vi "Autonomous Independent.vi"() -> ()   [LabVIEW 2017]
doc: "This VI is called when autonomous begins, and will automatically be terminated when autonomous ends. You can carry out timed or sensor driven robot movement independently without needing to return to the caller."
uses:
  <vilib>/Rock Robotics/WPI/Solenoid/WPI_SolenoidValue.ctl
  <vilib>/Rock Robotics/WPI/SafetyOutput/WPI_SafetyOutputConfigMenu.ctl
  <vilib>/Rock Robotics/WPI/Utilities/WPI_GetSetVariantRefNum.vi
  <vilib>/Rock Robotics/Network Tables/NT Read String.vi
  <vilib>/Rock Robotics/Network Tables/NT Write Numeric Array.vi
  <vilib>/Rock Robotics/WPI/Solenoid/WPI_SolenoidSetEnum.vi
  <vilib>/Rock Robotics/Network Tables/NT Read Numeric Array.vi
  <vilib>/Rock Robotics/Network Tables/NT Read Number.vi
  Robot Global Data.vi
  <vilib>/Rock Robotics/WPI/RobotDrive/WPI_RobotDriveArcadeDrive_Standard(NoSaturation).vi
panel:
  in  "Gear and B":dbl[](array[numeric])=[79.0, -39.5, 48.0, 160.0]
  in  "Drive Forward":dbl[](array[numeric])=[102.0, 0.0, 0.0, 0.0]
  in  "Station 3 Distances":dbl[](array[numeric])=[108.0, 10.0, -10.0, 20.0]
  in  "Station 1 Distances":dbl[](array[numeric])=[48.0, 24.0, -24.0, 96.0]
  in  "Station 2 Distances":dbl[](array[numeric])=[90.0, -48.0, 48.0, 120.0]
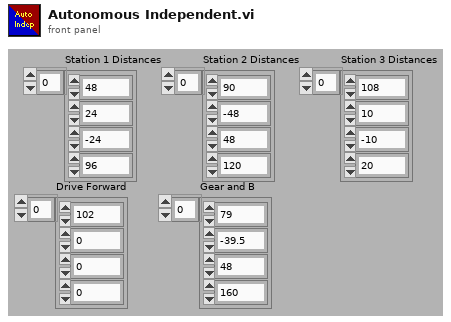
[diagram p1: front panel]
types:
  T1 = typedef "WPI_SolenoidValue.ctl" = enum16{"Off", "On", "Forward", "Reverse"}
  T2 = typedef "WPI_SolenoidDevRef.ctl" = cluster{"DevStatus":errorcluster, "Pneumatics Control Module":u8, "Forward Solenoid Channel":T3, "Reverse Solenoid Channel":T3}
  T3 = typedef "WPI_SolenoidChannel.ctl" = enum8{"Solenoid 0", "Solenoid 1", "Solenoid 2", "Solenoid 3", "Solenoid 4", "Solenoid 5", "Solenoid 6", "Solenoid 7", "Invalid"}
  T4 = typedef "WPI_JoystickDevRef.ctl" = cluster{"Device":T5}
  T5 = typedef "WPI_JoystickDeviceEnum.ctl" = enum16{"USB 0", "USB 1", "USB 2", "USB 3", "USB 4", "USB 5"}
  T6 = cluster{"Numeric Array":dbl[], "Numeric":dbl, "Numeric":dbl, "Numeric":dbl}
  T7 = cluster{"Numeric Array":dbl[], "Numeric":dbl, "Numeric":dbl}
  T8 = typedef "WPI_SafetyOutputConfigMenu.ctl" = enum16{"Enable", "Disable"}
  T9 = typedef "WPI_RobotDriveDevRef.ctl" = cluster{"DevStatus":errorcluster, "Motors[]":T10[], "Square Inputs":bool, "Max Output":dbl}
  T10 = typedef "WPI_MotorControlDeviceRef.ctl" = cluster{"DeviceStatus":errorcluster, "Type":T11, "PWM":cluster{"PWM Channel":T12, "DeadBand":T13}, "CAN":cluster{"Device Number":u8, "SetOutput VI Ref":variant, "GetOutput VI Ref":variant, "Enable VI Ref":variant, "Disable VI Ref":variant, "Data":variant}, "Invert":bool, "DIO PWM":cluster{"PWM \"Enable\" Channel":T12, "DIOChannel":T14, "PWM Rate":dbl}}
  T11 = typedef "WPI_MotorControlType.ctl" = enum16{"PWM", "CAN", "DIO PWM"}
  T12 = typedef "FPGA_DIOPWMChannel.ctl" = enum8{"PWM 0", "PWM 1", "PWM 2", "PWM 3", "PWM 4", "PWM 5", "PWM 6", "PWM 7", "PWM 8", "PWM 9", "PWM MXP 0", "PWM MXP 1", "PWM MXP 2", "PWM MXP 3", "PWM MXP 4", "PWM MXP 5", "PWM MXP 6", "PWM MXP 7", "PWM MXP 8", "PWM MXP 9", "Invalid"}
  T13 = typedef "WPI_PWMDeadband.ctl" = cluster{"Name":string, "maxPositivePwm":i32, "minPositivePwm":i32, "centerPwm":i32, "maxNegativePwm":i32, "minNegativePwm":i32, "angularRange":u16}
  T14 = typedef "FPGA_DIOChannel.ctl" = enum8{"DIO 0", "DIO 1", "DIO 2", "DIO 3", "DIO 4", "DIO 5", "DIO 6", "DIO 7", "DIO 8", "DIO 9", "DIO MXP 0", "DIO MXP 1", "DIO MXP 2", "DIO MXP 3", "DIO MXP 4", "DIO MXP 5", "DIO MXP 6", "DIO MXP 7", "DIO MXP 8", "DIO MXP 9", "DIO MXP 10", "DIO MXP 11", "DIO MXP 12", "DIO MXP 13", "DIO MXP 14", "DIO MXP 15", "SPI Port CS1", "SPI Port CS2", "SPI Port CS3", "SPI Port MISO", "SPI Port MOSI", "Invalid"}
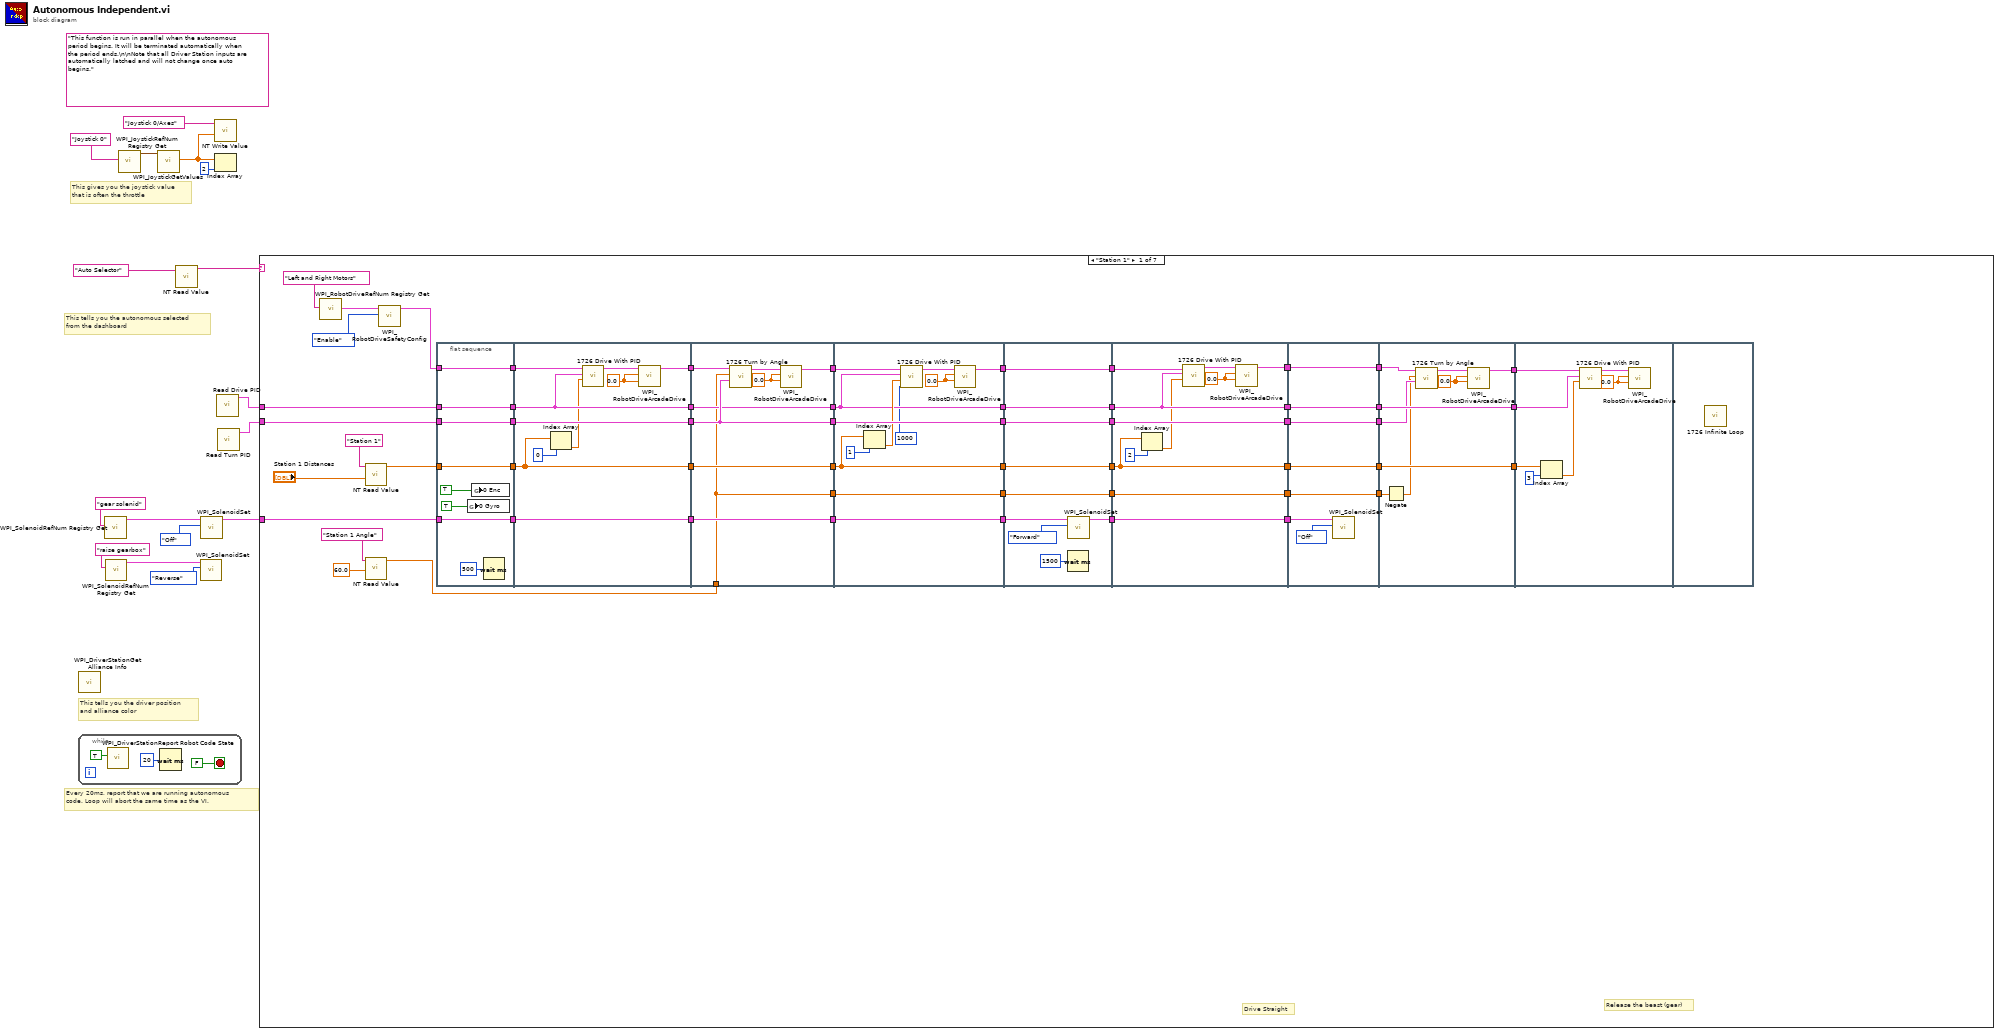
[diagram p0: block diagram]
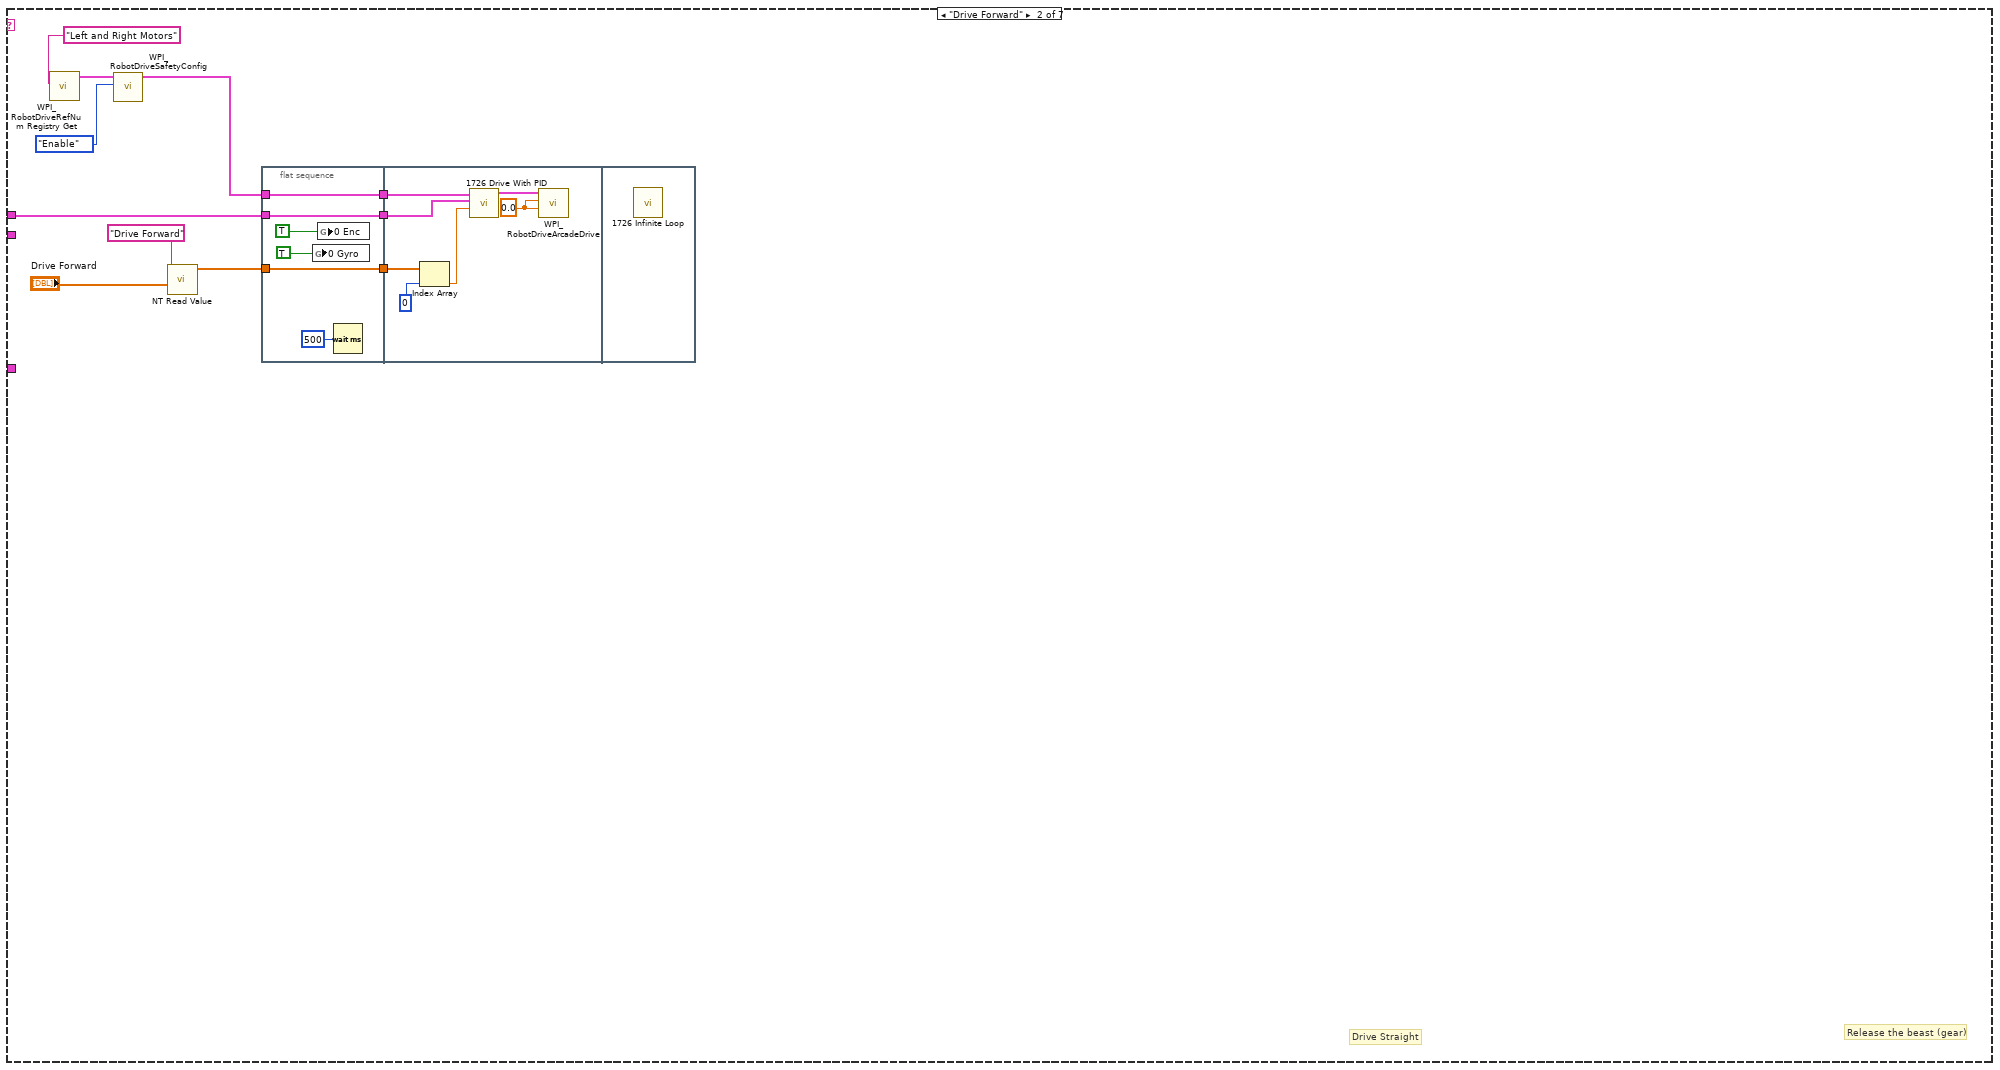
[diagram p2: hidden frame]
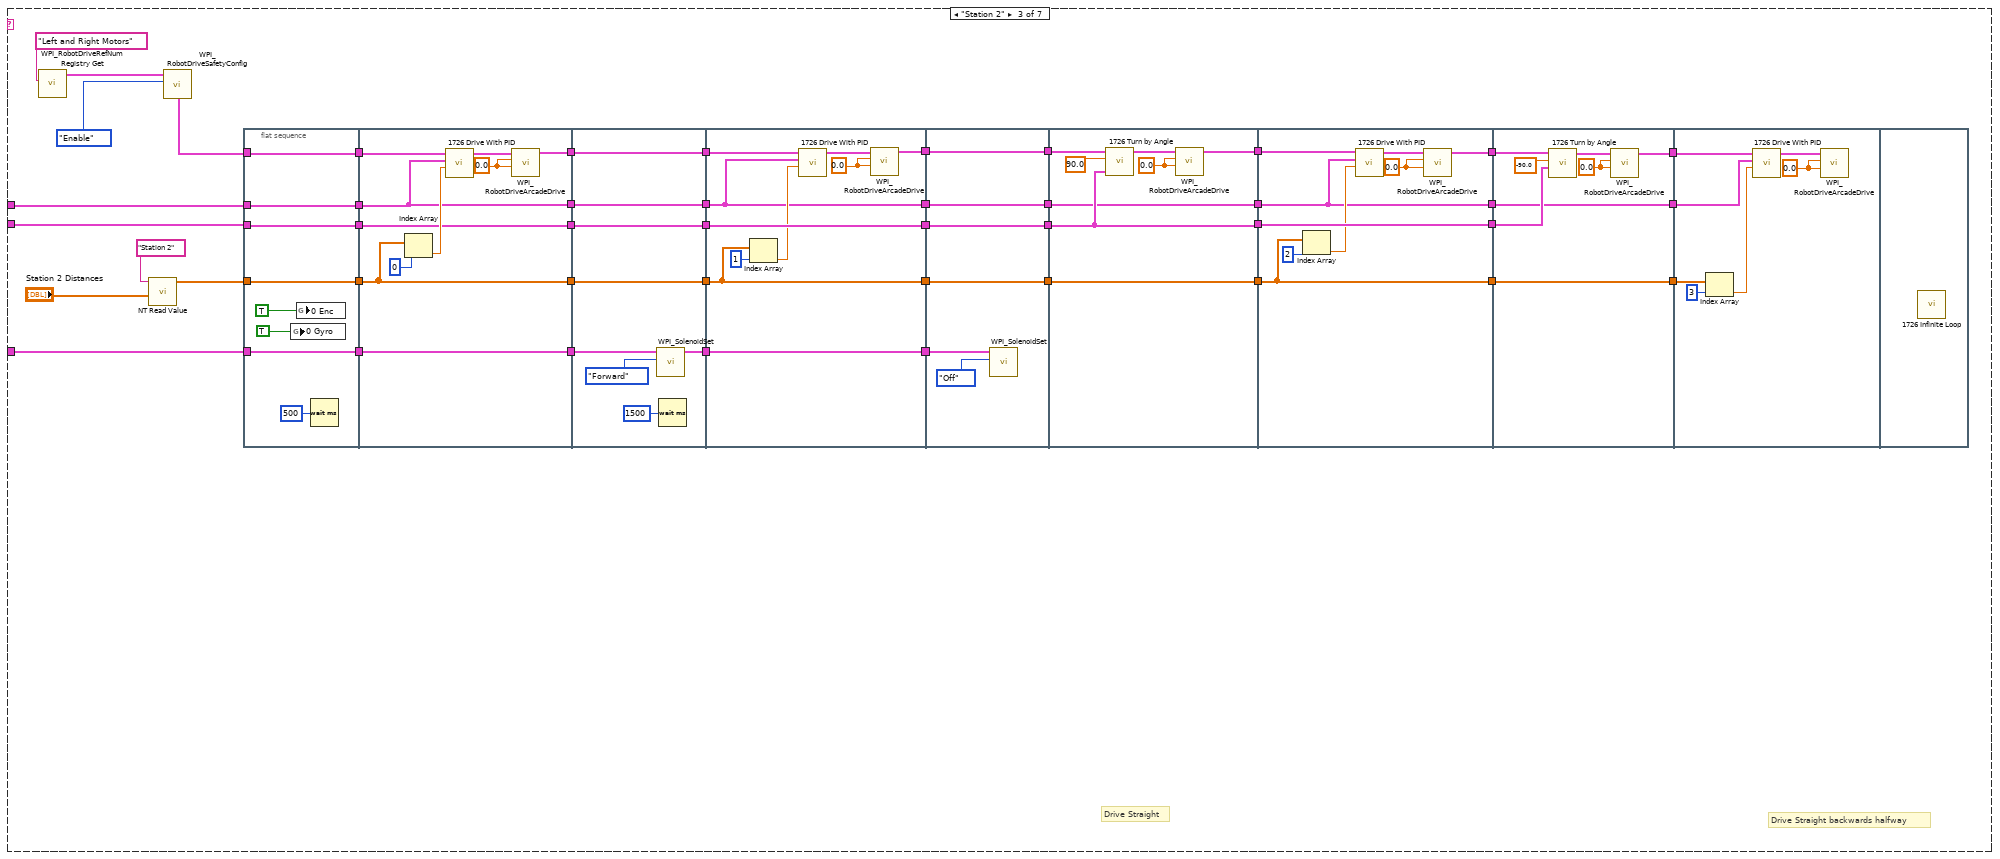
[diagram p3: hidden frame]
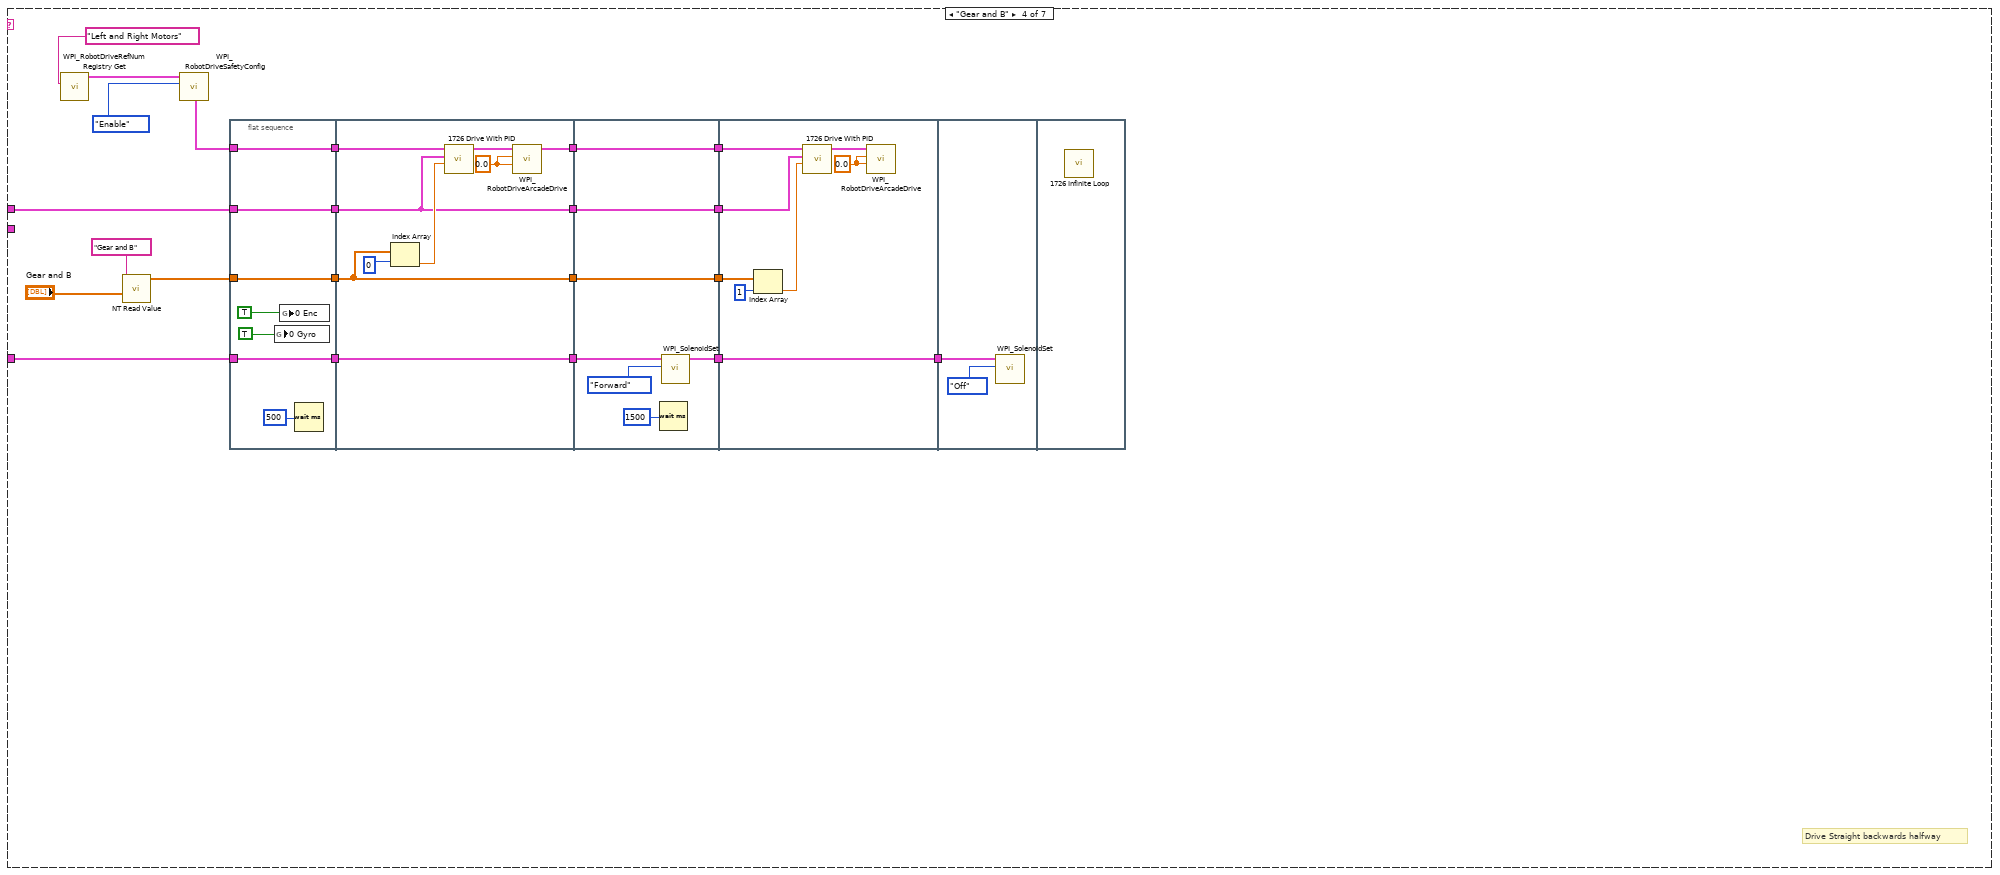
[diagram p4: hidden frame]
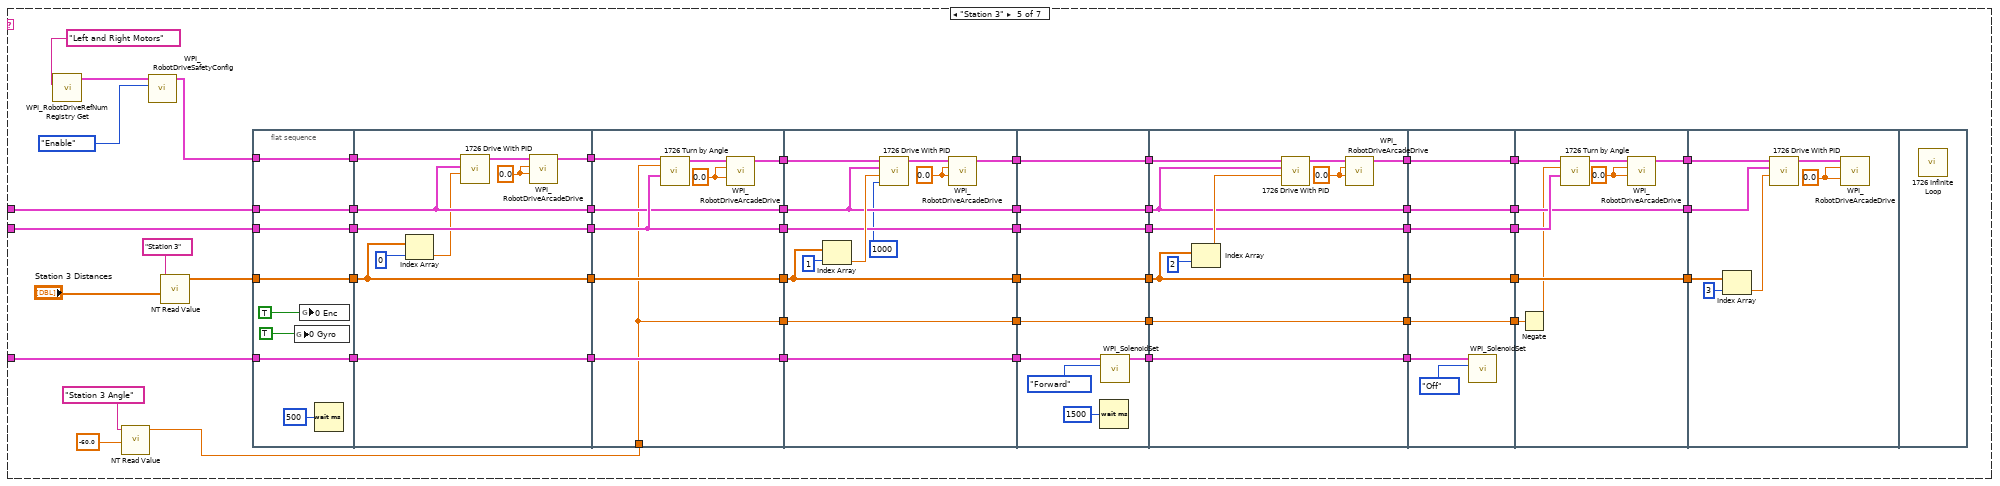
[diagram p5: hidden frame]
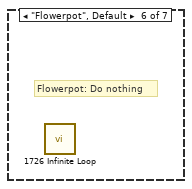
[diagram p6: hidden frame]
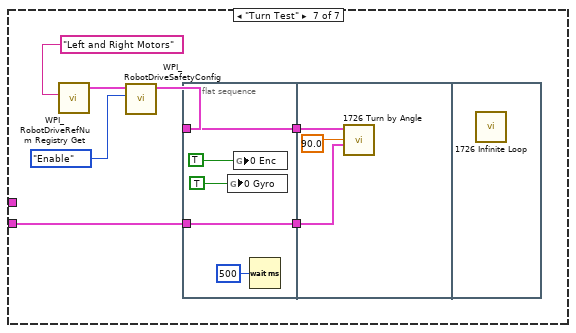
[diagram p7: hidden frame]
diagram:
  (unwired) "This function is run in parallel when the autonomous period begins. It will be terminated automatically when the period ends.\n\nNote that all Driver Station inputs are automatically latched and will not change once auto begins."
  # "This tells you the autonomous selected\nfrom the dashboard"
  # "Every 20ms, report that we are running autonomous\ncode. Loop will abort the same time as the VI."
  # "This gives you the joystick value\nthat is often the throttle"
  # "This tells you the driver position\nand alliance color"
  n1 = while {
    stop <- FALSE stop-if-true
    n2 = call <vilib>:"WPI_DriverStationReport Robot Code State.vi"("Autonomous"=TRUE) -> ()  [unwired: 10 in, 1 out]
    n3 = Wait (ms)(milliseconds to wait=u32 20) -> ()  [unwired: 1 out]
  }
  n4 = call <vilib>:"WPI_DriverStationGet Alliance Info.vi"() -> ()  [unwired: 12 out]
  n5 = call <vilib>:"WPI_SolenoidRefNum Registry Get.vi"("refnum name"="gear solenid") -> ("SolenoidDevRef"=w6:T2)  [unwired: 9 in, 1 out]
  n6 = call <vilib>:"WPI_SolenoidRefNum Registry Get.vi"("refnum name"="raise gearbox") -> ("SolenoidDevRef"=w3:T2)  [unwired: 9 in, 1 out]
  n7 = call <vilib>:"WPI_JoystickRefNum Registry Get.vi"("refnum name"="Joystick 0") -> ("JoystickDevRef"=w15:T4)  [unwired: 1 in, 9 out]
  n8 = call <vilib>:"WPI_JoystickGetValues.vi"("JoystickDevRef"=w15) -> ("Axes"=w11:dbl[])  [unwired: 6 in, 4 out]
  n9 = call-poly <vilib>:"NT Read Value.vi"("Name"="Auto Selector") -> ("String"=w12:string)  [unwired: 9 in, 1 out]
  n10 = call-poly <vilib>:"WPI_SolenoidSet.vi"("Value"=WPI_SolenoidValue."Reverse", "SolenoidDevRef"=w3) -> ()  [unwired: 8 in, 2 out]
  n11 = call-poly <vilib>:"WPI_SolenoidSet.vi"("Value"=WPI_SolenoidValue."Off", "SolenoidDevRef"=w6) -> ("SolenoidDevRef"=w5:T2)  [unwired: 8 in, 1 out]
  n12 = call-poly <vilib>:"NT Write Value.vi"("Numeric Array"=w11, "Name"="Joystick 0/Axes") -> ()  [unwired: 9 in, 1 out]
  n13 = Index Array(array=w11, index=2) -> ()  [unwired: 1 out]
  n14 = call "Read Drive PID.vi"() -> ("Cluster"=w2:T6)  [unwired: 11 in]
  n15 = call "Read Turn PID.vi"() -> ("Cluster"=w1:T7)  [unwired: 11 in]
  n16 = case shown="\"Station 1\"" w12 {
    tunnel: w1 -> [w48 _ w202 _ w383 _ w494]
    tunnel: w2 -> [w41 w163 w195 w310 w377 _ _]
    tunnel: w5 -> [w33 _ w186 w304 w368 _ _]
    frame "Station 1" {
      # "Release the beast (gear)"
      # "Drive Straight"
      n17 = call <vilib>:"WPI_RobotDriveRefNum Registry Get.vi"("refnum name"="Left and Right Motors") -> ("RobotDriveDevRef"=w64:T9)  [unwired: 1 in, 9 out]
      n18 = call-poly <vilib>:"NT Read Value.vi"("Default Value"="Station 1 Distances", "Name"="Station 1") -> ("Numeric Array"=w50:dbl[])  [unwired: 8 in, 1 out]
      n19 = call-poly <vilib>:"NT Read Value.vi"("Default Value"=60.0, "Name"="Station 1 Angle") -> ("Numeric"=w25:dbl)  [unwired: 8 in, 1 out]
      n20 = call <vilib>:"WPI_RobotDriveSafetyConfig.vi"("mode"=WPI_SafetyOutputConfigMenu."Enable", "RobotDriveDevRef"=w64) -> ("RobotDriveDevRef"=w62:T9)  [unwired: 8 in, 1 out]
      n21 = flat-sequence {
        tunnel: w50 -> [w78]
        tunnel: w33 -> [w79]
        tunnel: w62 -> [w80]
        tunnel: w48 -> [w81]
        tunnel: w41 -> [w82]
        tunnel: [w82] -> w32
        tunnel: [w81] -> w31
        tunnel: [w80] -> w30
        tunnel: [w79] -> w29
        tunnel: [w78] -> w28
        tunnel: [w92] -> w74
        tunnel: [w91] -> w73
        tunnel: [w90] -> w72
        tunnel: [w89] -> w47
        tunnel: [w88] -> w40
        tunnel: w32 -> [w88]
        tunnel: w31 -> [w89]
        tunnel: w30 -> [w86]
        tunnel: w29 -> [w90]
        tunnel: w28 -> [w91]
        tunnel: [w101] -> w71
        tunnel: [w100] -> w70
        tunnel: [w99] -> w61
        tunnel: [w98] -> w46
        tunnel: [w97] -> w38
        tunnel: w40 -> [w97]
        tunnel: w47 -> [w98]
        tunnel: w72 -> [w99]
        tunnel: w73 -> [w100]
        tunnel: w74 -> [w94]
        tunnel: w25 -> [w93]
        tunnel: [w93] -> w24
        tunnel: [w113] -> w69
        tunnel: [w111] -> w68
        tunnel: w71 -> [w110]
        tunnel: w70 -> [w111]
        tunnel: w61 -> [w109]
        tunnel: [w109] -> w60
        tunnel: w46 -> [w106]
        tunnel: [w106] -> w45
        tunnel: [w104] -> w39
        tunnel: w38 -> [w104]
        tunnel: w24 -> [w102]
        tunnel: [w102] -> w23
        tunnel: w69 -> [w122]
        tunnel: [w122] -> w59
        tunnel: w68 -> [w121]
        tunnel: [w121] -> w58
        tunnel: w60 -> [w119]
        tunnel: [w118] -> w57
        tunnel: w45 -> [w117]
        tunnel: [w117] -> w43
        tunnel: w39 -> [w116]
        tunnel: [w116] -> w37
        tunnel: w23 -> [w114]
        tunnel: [w114] -> w22
        tunnel: w59 -> [w132]
        tunnel: [w131] -> w56
        tunnel: w58 -> [w128]
        tunnel: w57 -> [w133]
        tunnel: [w133] -> w53
        tunnel: [w128] -> w52
        tunnel: [w126] -> w44
        tunnel: w43 -> [w126]
        tunnel: w37 -> [w125]
        tunnel: [w125] -> w36
        tunnel: w22 -> [w123]
        tunnel: [w123] -> w21
        tunnel: w56 -> [w140]
        tunnel: [w140] -> w55
        tunnel: [w139] -> w54
        tunnel: w53 -> [w137]
        tunnel: w52 -> [w139]
        tunnel: w44 -> [w136]
        tunnel: [w136] -> w42
        tunnel: w36 -> [w135]
        tunnel: [w135] -> w34
        tunnel: w21 -> [w134]
        tunnel: [w134] -> w20
        tunnel: [w149] -> w67
        tunnel: [w148] -> w66
        tunnel: [w147] -> w35
        tunnel: w34 -> [w147]
        tunnel: w42 -> [w144]
        tunnel: w54 -> [w148]
        tunnel: w55 -> [w145]
        tunnel: w20 -> [w142]
        tunnel: w67 -> [w154]
        tunnel: w66 -> [w152]
        tunnel: w35 -> [w150]
        frame #0 {
          n22 = global write "Robot Global Data.vi" "0 Gyro"(TRUE ("0 Gyro")) -> ()
          n23 = global write "Robot Global Data.vi" "0 Enc"(TRUE ("0 Enc")) -> ()
          n24 = Wait (ms)(milliseconds to wait=u32 500) -> ()  [unwired: 1 out]
        }
        frame #1 {
          w87 = 0.0 ("X axis value")
          n25 = Index Array(array=w91, index=0) -> (element=w83:dbl)
          n26 = call "1726 Drive With PID.vi"("RobotDriveDevRef in"=w86, "Tuning Parametres"=w88, "Target Distance"=w83) -> ("RobotDriveDevRef out"=w84:T9)  [unwired: 5 in, 2 out]
          n27 = call-poly <vilib>:"WPI_RobotDriveArcadeDrive.vi"("Y axis value"=w87, "X axis value"=w87, "RobotDriveDevRef"=w84) -> ("RobotDriveDevRef"=w92:T9)  [unwired: 6 in, 2 out]
        }
        frame #2 {
          w96 = 0.0 ("X axis value")
          n28 = call "1726 Turn by Angle.vi"("RobotDriveDevRef in"=w94, "Target Angle"=w93, "Tuning Parametres"=w98) -> ("RobotDriveDevRef out"=w95:T9)  [unwired: 5 in, 2 out]
          n29 = call-poly <vilib>:"WPI_RobotDriveArcadeDrive.vi"("Y axis value"=w96, "X axis value"=w96, "RobotDriveDevRef"=w95) -> ("RobotDriveDevRef"=w101:T9)  [unwired: 6 in, 2 out]
        }
        frame #3 {
          w108 = 0.0 ("X axis value")
          n30 = Index Array(array=w111, index=1) -> (element=w105:dbl)
          n31 = call "1726 Drive With PID.vi"("RobotDriveDevRef in"=w110, "Tuning Parametres"=w104, "Target Distance"=w105, "Timeout (ms)"=u32 1000) -> ("RobotDriveDevRef out"=w107:T9)  [unwired: 4 in, 2 out]
          n32 = call-poly <vilib>:"WPI_RobotDriveArcadeDrive.vi"("Y axis value"=w108, "X axis value"=w108, "RobotDriveDevRef"=w107) -> ("RobotDriveDevRef"=w113:T9)  [unwired: 6 in, 2 out]
        }
        frame #4 {
          n33 = Wait (ms)(milliseconds to wait=u32 1500) -> ()  [unwired: 1 out]
          n34 = call-poly <vilib>:"WPI_SolenoidSet.vi"("Value"=WPI_SolenoidValue."Forward", "SolenoidDevRef"=w119) -> ("SolenoidDevRef"=w118:T2)  [unwired: 8 in, 1 out]
        }
        frame #5 {
          w130 = 0.0 ("X axis value")
          n35 = Index Array(array=w128, index=2) -> (element=w124:dbl)
          n36 = call "1726 Drive With PID.vi"("RobotDriveDevRef in"=w132, "Tuning Parametres"=w125, "Target Distance"=w124) -> ("RobotDriveDevRef out"=w127:T9)  [unwired: 5 in, 2 out]
          n37 = call-poly <vilib>:"WPI_RobotDriveArcadeDrive.vi"("Y axis value"=w130, "X axis value"=w130, "RobotDriveDevRef"=w127) -> ("RobotDriveDevRef"=w131:T9)  [unwired: 6 in, 2 out]
        }
        frame #6 {
          n38 = call-poly <vilib>:"WPI_SolenoidSet.vi"("Value"=WPI_SolenoidValue."Off", "SolenoidDevRef"=w137) -> ()  [unwired: 8 in, 2 out]
        }
        frame #7 {
          w143 = 0.0 ("X axis value")
          n39 = Negate(x=w142) -> (-x=w141:dbl)
          n40 = call "1726 Turn by Angle.vi"("RobotDriveDevRef in"=w145, "Target Angle"=w141, "Tuning Parametres"=w144) -> ("RobotDriveDevRef out"=w146:T9)  [unwired: 5 in, 2 out]
          n41 = call-poly <vilib>:"WPI_RobotDriveArcadeDrive.vi"("Y axis value"=w143, "X axis value"=w143, "RobotDriveDevRef"=w146) -> ("RobotDriveDevRef"=w149:T9)  [unwired: 6 in, 2 out]
        }
        frame #8 {
          w156 = 0.0 ("X axis value")
          n42 = Index Array(array=w152, index=3) -> (element=w151:dbl)
          n43 = call "1726 Drive With PID.vi"("RobotDriveDevRef in"=w154, "Tuning Parametres"=w150, "Target Distance"=w151) -> ("RobotDriveDevRef out"=w155:T9)  [unwired: 5 in, 2 out]
          n44 = call-poly <vilib>:"WPI_RobotDriveArcadeDrive.vi"("Y axis value"=w156, "X axis value"=w156, "RobotDriveDevRef"=w155) -> ()  [unwired: 6 in, 3 out]
        }
        frame #9 {
          n45 = call "1726 Infinite Loop.vi"() -> ()  [unwired: 12 in]
        }
      }
    }
    frame "Drive Forward" {
      # "Release the beast (gear)"
      # "Drive Straight"
      n46 = call <vilib>:"WPI_RobotDriveRefNum Registry Get.vi"("refnum name"="Left and Right Motors") -> ("RobotDriveDevRef"=w166:T9)  [unwired: 1 in, 9 out]
      n47 = call <vilib>:"WPI_RobotDriveSafetyConfig.vi"("mode"=WPI_SafetyOutputConfigMenu."Enable", "RobotDriveDevRef"=w166) -> ("RobotDriveDevRef"=w164:T9)  [unwired: 8 in, 1 out]
      n48 = call-poly <vilib>:"NT Read Value.vi"("Default Value"="Drive Forward", "Name"="Drive Forward") -> ("Numeric Array"=w160:dbl[])  [unwired: 8 in, 1 out]
      n49 = flat-sequence {
        tunnel: w160 -> [w171]
        tunnel: w164 -> [w172]
        tunnel: w163 -> [w173]
        tunnel: [w173] -> w159
        tunnel: [w172] -> w158
        tunnel: [w171] -> w157
        tunnel: w159 -> [w174]
        tunnel: w158 -> [w178]
        tunnel: w157 -> [w180]
        frame #0 {
          n50 = global write "Robot Global Data.vi" "0 Gyro"(TRUE ("0 Gyro")) -> ()
          n51 = global write "Robot Global Data.vi" "0 Enc"(TRUE ("0 Enc")) -> ()
          n52 = Wait (ms)(milliseconds to wait=u32 500) -> ()  [unwired: 1 out]
        }
        frame #1 {
          w179 = 0.0 ("X axis value")
          n53 = Index Array(array=w180, index=0) -> (element=w175:dbl)
          n54 = call "1726 Drive With PID.vi"("RobotDriveDevRef in"=w178, "Tuning Parametres"=w174, "Target Distance"=w175) -> ("RobotDriveDevRef out"=w176:T9)  [unwired: 5 in, 2 out]
          n55 = call-poly <vilib>:"WPI_RobotDriveArcadeDrive.vi"("Y axis value"=w179, "X axis value"=w179, "RobotDriveDevRef"=w176) -> ()  [unwired: 6 in, 3 out]
        }
        frame #2 {
          n56 = call "1726 Infinite Loop.vi"() -> ()  [unwired: 12 in]
        }
      }
    }
    frame "Station 2" {
      # "Drive Straight backwards halfway"
      # "Drive Straight"
      n57 = call <vilib>:"WPI_RobotDriveRefNum Registry Get.vi"("refnum name"="Left and Right Motors") -> ("RobotDriveDevRef"=w224:T9)  [unwired: 1 in, 9 out]
      n58 = call-poly <vilib>:"NT Read Value.vi"("Default Value"="Station 2 Distances", "Name"="Station 2") -> ("Numeric Array"=w205:dbl[])  [unwired: 8 in, 1 out]
      n59 = call <vilib>:"WPI_RobotDriveSafetyConfig.vi"("mode"=WPI_SafetyOutputConfigMenu."Enable", "RobotDriveDevRef"=w224) -> ("RobotDriveDevRef"=w223:T9)  [unwired: 8 in, 1 out]
      n60 = flat-sequence {
        tunnel: w223 -> [w229]
        tunnel: w205 -> [w230]
        tunnel: w186 -> [w231]
        tunnel: w202 -> [w232]
        tunnel: w195 -> [w233]
        tunnel: [w233] -> w185
        tunnel: [w232] -> w184
        tunnel: [w231] -> w183
        tunnel: [w230] -> w182
        tunnel: [w229] -> w181
        tunnel: [w240] -> w221
        tunnel: [w237] -> w215
        tunnel: [w236] -> w209
        tunnel: [w235] -> w200
        tunnel: [w234] -> w194
        tunnel: w185 -> [w234]
        tunnel: w184 -> [w235]
        tunnel: w183 -> [w236]
        tunnel: w182 -> [w237]
        tunnel: w181 -> [w241]
        tunnel: w221 -> [w251]
        tunnel: [w251] -> w220
        tunnel: w215 -> [w249]
        tunnel: [w249] -> w214
        tunnel: w209 -> [w247]
        tunnel: [w246] -> w208
        tunnel: [w245] -> w201
        tunnel: w200 -> [w245]
        tunnel: w194 -> [w244]
        tunnel: [w244] -> w193
        tunnel: w220 -> [w260]
        tunnel: [w259] -> w219
        tunnel: w214 -> [w257]
        tunnel: [w257] -> w213
        tunnel: w208 -> [w256]
        tunnel: [w256] -> w207
        tunnel: w201 -> [w254]
        tunnel: [w254] -> w198
        tunnel: w193 -> [w252]
        tunnel: [w252] -> w191
        tunnel: w219 -> [w267]
        tunnel: [w267] -> w218
        tunnel: w213 -> [w266]
        tunnel: [w266] -> w212
        tunnel: w207 -> [w264]
        tunnel: [w263] -> w199
        tunnel: w198 -> [w263]
        tunnel: w191 -> [w262]
        tunnel: [w262] -> w190
        tunnel: w218 -> [w275]
        tunnel: [w274] -> w204
        tunnel: w212 -> [w273]
        tunnel: [w273] -> w203
        tunnel: w199 -> [w271]
        tunnel: [w271] -> w196
        tunnel: w190 -> [w268]
        tunnel: [w268] -> w189
        tunnel: [w284] -> w217
        tunnel: [w282] -> w211
        tunnel: [w279] -> w197
        tunnel: w204 -> [w278]
        tunnel: w203 -> [w282]
        tunnel: w196 -> [w279]
        tunnel: w189 -> [w276]
        tunnel: [w276] -> w188
        tunnel: [w292] -> w216
        tunnel: [w291] -> w210
        tunnel: w217 -> [w290]
        tunnel: w211 -> [w291]
        tunnel: w197 -> [w288]
        tunnel: w188 -> [w285]
        tunnel: [w285] -> w187
        tunnel: w216 -> [w297]
        tunnel: w210 -> [w295]
        tunnel: w187 -> [w293]
        frame #0 {
          n61 = global write "Robot Global Data.vi" "0 Gyro"(TRUE ("0 Gyro")) -> ()
          n62 = global write "Robot Global Data.vi" "0 Enc"(TRUE ("0 Enc")) -> ()
          n63 = Wait (ms)(milliseconds to wait=u32 500) -> ()  [unwired: 1 out]
        }
        frame #1 {
          w243 = 0.0 ("X axis value")
          n64 = Index Array(array=w237, index=0) -> (element=w238:dbl)
          n65 = call "1726 Drive With PID.vi"("RobotDriveDevRef in"=w241, "Tuning Parametres"=w234, "Target Distance"=w238) -> ("RobotDriveDevRef out"=w242:T9)  [unwired: 5 in, 2 out]
          n66 = call-poly <vilib>:"WPI_RobotDriveArcadeDrive.vi"("Y axis value"=w243, "X axis value"=w243, "RobotDriveDevRef"=w242) -> ("RobotDriveDevRef"=w240:T9)  [unwired: 6 in, 2 out]
        }
        frame #2 {
          n67 = call-poly <vilib>:"WPI_SolenoidSet.vi"("Value"=WPI_SolenoidValue."Forward", "SolenoidDevRef"=w247) -> ("SolenoidDevRef"=w246:T2)  [unwired: 8 in, 1 out]
          n68 = Wait (ms)(milliseconds to wait=u32 1500) -> ()  [unwired: 1 out]
        }
        frame #3 {
          w261 = 0.0 ("X axis value")
          n69 = Index Array(array=w257, index=1) -> (element=w253:dbl)
          n70 = call "1726 Drive With PID.vi"("RobotDriveDevRef in"=w260, "Tuning Parametres"=w252, "Target Distance"=w253) -> ("RobotDriveDevRef out"=w255:T9)  [unwired: 5 in, 2 out]
          n71 = call-poly <vilib>:"WPI_RobotDriveArcadeDrive.vi"("Y axis value"=w261, "X axis value"=w261, "RobotDriveDevRef"=w255) -> ("RobotDriveDevRef"=w259:T9)  [unwired: 6 in, 2 out]
        }
        frame #4 {
          n72 = call-poly <vilib>:"WPI_SolenoidSet.vi"("Value"=WPI_SolenoidValue."Off", "SolenoidDevRef"=w264) -> ()  [unwired: 8 in, 2 out]
        }
        frame #5 {
          w269 = 0.0 ("X axis value")
          n73 = call "1726 Turn by Angle.vi"("RobotDriveDevRef in"=w275, "Target Angle"=90.0, "Tuning Parametres"=w271) -> ("RobotDriveDevRef out"=w272:T9)  [unwired: 5 in, 2 out]
          n74 = call-poly <vilib>:"WPI_RobotDriveArcadeDrive.vi"("Y axis value"=w269, "X axis value"=w269, "RobotDriveDevRef"=w272) -> ("RobotDriveDevRef"=w274:T9)  [unwired: 6 in, 2 out]
        }
        frame #6 {
          w280 = 0.0 ("X axis value")
          n75 = Index Array(array=w282, index=2) -> (element=w277:dbl)
          n76 = call "1726 Drive With PID.vi"("RobotDriveDevRef in"=w278, "Tuning Parametres"=w276, "Target Distance"=w277) -> ("RobotDriveDevRef out"=w281:T9)  [unwired: 5 in, 2 out]
          n77 = call-poly <vilib>:"WPI_RobotDriveArcadeDrive.vi"("Y axis value"=w280, "X axis value"=w280, "RobotDriveDevRef"=w281) -> ("RobotDriveDevRef"=w284:T9)  [unwired: 6 in, 2 out]
        }
        frame #7 {
          w286 = 0.0 ("X axis value")
          n78 = call "1726 Turn by Angle.vi"("RobotDriveDevRef in"=w290, "Target Angle"=-90.0, "Tuning Parametres"=w288) -> ("RobotDriveDevRef out"=w289:T9)  [unwired: 5 in, 2 out]
          n79 = call-poly <vilib>:"WPI_RobotDriveArcadeDrive.vi"("Y axis value"=w286, "X axis value"=w286, "RobotDriveDevRef"=w289) -> ("RobotDriveDevRef"=w292:T9)  [unwired: 6 in, 2 out]
        }
        frame #8 {
          w299 = 0.0 ("X axis value")
          n80 = Index Array(array=w295, index=3) -> (element=w294:dbl)
          n81 = call "1726 Drive With PID.vi"("RobotDriveDevRef in"=w297, "Tuning Parametres"=w293, "Target Distance"=w294) -> ("RobotDriveDevRef out"=w298:T9)  [unwired: 5 in, 2 out]
          n82 = call-poly <vilib>:"WPI_RobotDriveArcadeDrive.vi"("Y axis value"=w299, "X axis value"=w299, "RobotDriveDevRef"=w298) -> ()  [unwired: 6 in, 3 out]
        }
        frame #9 {
          n83 = call "1726 Infinite Loop.vi"() -> ()  [unwired: 12 in]
        }
      }
    }
    frame "Gear and B" {
      # "Drive Straight backwards halfway"
      n84 = call <vilib>:"WPI_RobotDriveRefNum Registry Get.vi"("refnum name"="Left and Right Motors") -> ("RobotDriveDevRef"=w320:T9)  [unwired: 1 in, 9 out]
      n85 = call-poly <vilib>:"NT Read Value.vi"("Default Value"="Gear and B", "Name"="Gear and B") -> ("Numeric Array"=w305:dbl[])  [unwired: 8 in, 1 out]
      n86 = call <vilib>:"WPI_RobotDriveSafetyConfig.vi"("mode"=WPI_SafetyOutputConfigMenu."Enable", "RobotDriveDevRef"=w320) -> ("RobotDriveDevRef"=w319:T9)  [unwired: 8 in, 1 out]
      n87 = flat-sequence {
        tunnel: w319 -> [w325]
        tunnel: w305 -> [w326]
        tunnel: w304 -> [w327]
        tunnel: w310 -> [w328]
        tunnel: [w328] -> w303
        tunnel: [w327] -> w302
        tunnel: [w326] -> w301
        tunnel: [w325] -> w300
        tunnel: [w334] -> w317
        tunnel: [w332] -> w315
        tunnel: [w331] -> w313
        tunnel: [w329] -> w309
        tunnel: w303 -> [w329]
        tunnel: w302 -> [w331]
        tunnel: w301 -> [w332]
        tunnel: w300 -> [w335]
        tunnel: w317 -> [w344]
        tunnel: [w344] -> w316
        tunnel: w315 -> [w342]
        tunnel: [w342] -> w314
        tunnel: w313 -> [w340]
        tunnel: [w339] -> w312
        tunnel: w309 -> [w338]
        tunnel: [w338] -> w308
        tunnel: w316 -> [w351]
        tunnel: w314 -> [w349]
        tunnel: w312 -> [w348]
        tunnel: [w348] -> w311
        tunnel: w308 -> [w345]
        tunnel: w311 -> [w353]
        frame #0 {
          n88 = global write "Robot Global Data.vi" "0 Gyro"(TRUE ("0 Gyro")) -> ()
          n89 = global write "Robot Global Data.vi" "0 Enc"(TRUE ("0 Enc")) -> ()
          n90 = Wait (ms)(milliseconds to wait=u32 500) -> ()  [unwired: 1 out]
        }
        frame #1 {
          w337 = 0.0 ("X axis value")
          n91 = Index Array(array=w332, index=0) -> (element=w330:dbl)
          n92 = call "1726 Drive With PID.vi"("RobotDriveDevRef in"=w335, "Tuning Parametres"=w329, "Target Distance"=w330) -> ("RobotDriveDevRef out"=w336:T9)  [unwired: 5 in, 2 out]
          n93 = call-poly <vilib>:"WPI_RobotDriveArcadeDrive.vi"("Y axis value"=w337, "X axis value"=w337, "RobotDriveDevRef"=w336) -> ("RobotDriveDevRef"=w334:T9)  [unwired: 6 in, 2 out]
        }
        frame #2 {
          n94 = Wait (ms)(milliseconds to wait=u32 1500) -> ()  [unwired: 1 out]
          n95 = call-poly <vilib>:"WPI_SolenoidSet.vi"("Value"=WPI_SolenoidValue."Forward", "SolenoidDevRef"=w340) -> ("SolenoidDevRef"=w339:T2)  [unwired: 8 in, 1 out]
        }
        frame #3 {
          w352 = 0.0 ("X axis value")
          n96 = Index Array(array=w349, index=1) -> (element=w346:dbl)
          n97 = call "1726 Drive With PID.vi"("RobotDriveDevRef in"=w351, "Tuning Parametres"=w345, "Target Distance"=w346) -> ("RobotDriveDevRef out"=w347:T9)  [unwired: 5 in, 2 out]
          n98 = call-poly <vilib>:"WPI_RobotDriveArcadeDrive.vi"("Y axis value"=w352, "X axis value"=w352, "RobotDriveDevRef"=w347) -> ()  [unwired: 6 in, 3 out]
        }
        frame #4 {
          n99 = call-poly <vilib>:"WPI_SolenoidSet.vi"("Value"=WPI_SolenoidValue."Off", "SolenoidDevRef"=w353) -> ()  [unwired: 8 in, 2 out]
        }
        frame #5 {
          n100 = call "1726 Infinite Loop.vi"() -> ()  [unwired: 12 in]
        }
      }
    }
    frame "Station 3" {
      n101 = call <vilib>:"WPI_RobotDriveRefNum Registry Get.vi"("refnum name"="Left and Right Motors") -> ("RobotDriveDevRef"=w389:T9)  [unwired: 1 in, 9 out]
      n102 = call-poly <vilib>:"NT Read Value.vi"("Default Value"=-60.0, "Name"="Station 3 Angle") -> ("Numeric"=w360:dbl)  [unwired: 8 in, 1 out]
      n103 = call <vilib>:"WPI_RobotDriveSafetyConfig.vi"("mode"=WPI_SafetyOutputConfigMenu."Enable", "RobotDriveDevRef"=w389) -> ("RobotDriveDevRef"=w387:T9)  [unwired: 8 in, 1 out]
      n104 = call-poly <vilib>:"NT Read Value.vi"("Default Value"="Station 3 Distances", "Name"="Station 3") -> ("Numeric Array"=w385:dbl[])  [unwired: 8 in, 1 out]
      n105 = flat-sequence {
        tunnel: w385 -> [w413]
        tunnel: w368 -> [w414]
        tunnel: w387 -> [w415]
        tunnel: w383 -> [w416]
        tunnel: w377 -> [w417]
        tunnel: [w417] -> w367
        tunnel: [w416] -> w366
        tunnel: [w415] -> w365
        tunnel: [w414] -> w364
        tunnel: [w413] -> w363
        tunnel: [w427] -> w409
        tunnel: [w426] -> w408
        tunnel: [w425] -> w407
        tunnel: [w424] -> w384
        tunnel: [w423] -> w376
        tunnel: w367 -> [w423]
        tunnel: w366 -> [w424]
        tunnel: w365 -> [w421]
        tunnel: w364 -> [w425]
        tunnel: w363 -> [w426]
        tunnel: [w436] -> w406
        tunnel: [w435] -> w405
        tunnel: [w434] -> w404
        tunnel: [w433] -> w381
        tunnel: [w432] -> w374
        tunnel: w376 -> [w432]
        tunnel: w384 -> [w433]
        tunnel: w407 -> [w434]
        tunnel: w408 -> [w435]
        tunnel: w409 -> [w430]
        tunnel: w360 -> [w428]
        tunnel: [w428] -> w359
        tunnel: [w448] -> w403
        tunnel: [w445] -> w402
        tunnel: w406 -> [w444]
        tunnel: w405 -> [w445]
        tunnel: w404 -> [w443]
        tunnel: [w443] -> w401
        tunnel: [w440] -> w382
        tunnel: w381 -> [w440]
        tunnel: [w439] -> w375
        tunnel: w374 -> [w439]
        tunnel: w359 -> [w437]
        tunnel: [w437] -> w358
        tunnel: w403 -> [w457]
        tunnel: [w457] -> w400
        tunnel: w402 -> [w456]
        tunnel: [w456] -> w399
        tunnel: w401 -> [w454]
        tunnel: [w453] -> w398
        tunnel: w382 -> [w452]
        tunnel: [w452] -> w378
        tunnel: w375 -> [w451]
        tunnel: [w451] -> w373
        tunnel: w358 -> [w449]
        tunnel: [w449] -> w357
        tunnel: w400 -> [w467]
        tunnel: [w466] -> w397
        tunnel: w399 -> [w462]
        tunnel: w398 -> [w468]
        tunnel: [w468] -> w396
        tunnel: [w462] -> w395
        tunnel: [w460] -> w379
        tunnel: w378 -> [w460]
        tunnel: w373 -> [w459]
        tunnel: [w459] -> w372
        tunnel: w357 -> [w458]
        tunnel: [w458] -> w356
        tunnel: w397 -> [w475]
        tunnel: [w475] -> w394
        tunnel: [w474] -> w393
        tunnel: w396 -> [w472]
        tunnel: w395 -> [w474]
        tunnel: [w471] -> w380
        tunnel: w379 -> [w471]
        tunnel: w372 -> [w470]
        tunnel: [w470] -> w370
        tunnel: w356 -> [w469]
        tunnel: [w469] -> w355
        tunnel: w394 -> [w482]
        tunnel: [w483] -> w392
        tunnel: w393 -> [w484]
        tunnel: [w484] -> w391
        tunnel: w380 -> [w480]
        tunnel: [w479] -> w371
        tunnel: w370 -> [w479]
        tunnel: w355 -> [w477]
        tunnel: w371 -> [w485]
        tunnel: w391 -> [w487]
        tunnel: w392 -> [w490]
        frame #0 {
          n106 = global write "Robot Global Data.vi" "0 Gyro"(TRUE ("0 Gyro")) -> ()
          n107 = global write "Robot Global Data.vi" "0 Enc"(TRUE ("0 Enc")) -> ()
          n108 = Wait (ms)(milliseconds to wait=u32 500) -> ()  [unwired: 1 out]
        }
        frame #1 {
          w422 = 0.0 ("X axis value")
          n109 = Index Array(array=w426, index=0) -> (element=w419:dbl)
          n110 = call "1726 Drive With PID.vi"("RobotDriveDevRef in"=w421, "Tuning Parametres"=w423, "Target Distance"=w419) -> ("RobotDriveDevRef out"=w418:T9)  [unwired: 5 in, 2 out]
          n111 = call-poly <vilib>:"WPI_RobotDriveArcadeDrive.vi"("Y axis value"=w422, "X axis value"=w422, "RobotDriveDevRef"=w418) -> ("RobotDriveDevRef"=w427:T9)  [unwired: 6 in, 2 out]
        }
        frame #2 {
          w431 = 0.0 ("X axis value")
          n112 = call "1726 Turn by Angle.vi"("RobotDriveDevRef in"=w430, "Target Angle"=w428, "Tuning Parametres"=w433) -> ("RobotDriveDevRef out"=w429:T9)  [unwired: 5 in, 2 out]
          n113 = call-poly <vilib>:"WPI_RobotDriveArcadeDrive.vi"("Y axis value"=w431, "X axis value"=w431, "RobotDriveDevRef"=w429) -> ("RobotDriveDevRef"=w436:T9)  [unwired: 6 in, 2 out]
        }
        frame #3 {
          w442 = 0.0 ("X axis value")
          n114 = Index Array(array=w445, index=1) -> (element=w446:dbl)
          n115 = call "1726 Drive With PID.vi"("RobotDriveDevRef in"=w444, "Tuning Parametres"=w439, "Target Distance"=w446, "Timeout (ms)"=u32 1000) -> ("RobotDriveDevRef out"=w441:T9)  [unwired: 4 in, 2 out]
          n116 = call-poly <vilib>:"WPI_RobotDriveArcadeDrive.vi"("Y axis value"=w442, "X axis value"=w442, "RobotDriveDevRef"=w441) -> ("RobotDriveDevRef"=w448:T9)  [unwired: 6 in, 2 out]
        }
        frame #4 {
          n117 = Wait (ms)(milliseconds to wait=u32 1500) -> ()  [unwired: 1 out]
          n118 = call-poly <vilib>:"WPI_SolenoidSet.vi"("Value"=WPI_SolenoidValue."Forward", "SolenoidDevRef"=w454) -> ("SolenoidDevRef"=w453:T2)  [unwired: 8 in, 1 out]
        }
        frame #5 {
          w465 = 0.0 ("X axis value")
          n119 = Index Array(array=w462, index=2) -> (element=w463:dbl)
          n120 = call "1726 Drive With PID.vi"("RobotDriveDevRef in"=w467, "Tuning Parametres"=w459, "Target Distance"=w463) -> ("RobotDriveDevRef out"=w461:T9)  [unwired: 5 in, 2 out]
          n121 = call-poly <vilib>:"WPI_RobotDriveArcadeDrive.vi"("Y axis value"=w465, "X axis value"=w465, "RobotDriveDevRef"=w461) -> ("RobotDriveDevRef"=w466:T9)  [unwired: 6 in, 2 out]
        }
        frame #6 {
          n122 = call-poly <vilib>:"WPI_SolenoidSet.vi"("Value"=WPI_SolenoidValue."Off", "SolenoidDevRef"=w472) -> ()  [unwired: 8 in, 2 out]
        }
        frame #7 {
          w478 = 0.0 ("X axis value")
          n123 = Negate(x=w477) -> (-x=w476:dbl)
          n124 = call "1726 Turn by Angle.vi"("RobotDriveDevRef in"=w482, "Target Angle"=w476, "Tuning Parametres"=w480) -> ("RobotDriveDevRef out"=w481:T9)  [unwired: 5 in, 2 out]
          n125 = call-poly <vilib>:"WPI_RobotDriveArcadeDrive.vi"("Y axis value"=w478, "X axis value"=w478, "RobotDriveDevRef"=w481) -> ("RobotDriveDevRef"=w483:T9)  [unwired: 6 in, 2 out]
        }
        frame #8 {
          w491 = 0.0 ("X axis value")
          n126 = Index Array(array=w487, index=3) -> (element=w488:dbl)
          n127 = call "1726 Drive With PID.vi"("RobotDriveDevRef in"=w490, "Tuning Parametres"=w485, "Target Distance"=w488) -> ("RobotDriveDevRef out"=w486:T9)  [unwired: 5 in, 2 out]
          n128 = call-poly <vilib>:"WPI_RobotDriveArcadeDrive.vi"("Y axis value"=w491, "X axis value"=w491, "RobotDriveDevRef"=w486) -> ()  [unwired: 6 in, 3 out]
        }
        frame #9 {
          n129 = call "1726 Infinite Loop.vi"() -> ()  [unwired: 12 in]
        }
      }
    }
    frame "Flowerpot", Default {
      # "Flowerpot: Do nothing"
      n130 = call "1726 Infinite Loop.vi"() -> ()  [unwired: 12 in]
    }
    frame "Turn Test" {
      n131 = call <vilib>:"WPI_RobotDriveRefNum Registry Get.vi"("refnum name"="Left and Right Motors") -> ("RobotDriveDevRef"=w497:T9)  [unwired: 1 in, 9 out]
      n132 = call <vilib>:"WPI_RobotDriveSafetyConfig.vi"("mode"=WPI_SafetyOutputConfigMenu."Enable", "RobotDriveDevRef"=w497) -> ("RobotDriveDevRef"=w495:T9)  [unwired: 8 in, 1 out]
      n133 = flat-sequence {
        tunnel: w494 -> [w502]
        tunnel: w495 -> [w503]
        tunnel: [w503] -> w493
        tunnel: [w502] -> w492
        tunnel: w493 -> [w506]
        tunnel: w492 -> [w504]
        frame #0 {
          n134 = global write "Robot Global Data.vi" "0 Gyro"(TRUE ("0 Gyro")) -> ()
          n135 = global write "Robot Global Data.vi" "0 Enc"(TRUE ("0 Enc")) -> ()
          n136 = Wait (ms)(milliseconds to wait=u32 500) -> ()  [unwired: 1 out]
        }
        frame #1 {
          n137 = call "1726 Turn by Angle.vi"("RobotDriveDevRef in"=w506, "Target Angle"=90.0, "Tuning Parametres"=w504) -> ()  [unwired: 5 in, 3 out]
        }
        frame #2 {
          n138 = call "1726 Infinite Loop.vi"() -> ()  [unwired: 12 in]
        }
      }
    }
  }
